vi "Apply on Cell.vi"(8 "error in":errorcluster, 10 "Cell":refnum<class "Cell.lvclass">, 11 "Cell View Alternating Back Color in":refnum<class "Cell View Alternating Back Color.lvclass">) -> (0 "error out":errorcluster, 3 "Cell View Alternating Back Color out":refnum<class "Cell View Alternating Back Color.lvclass">)   [LabVIEW 2024, in "SourceGrid.lvlib" / "Cell View Alternating Back Color.lvclass"]
uses:
  Cell View Alternating Back Color.lvclass
  Cells/Cell/Cell.lvclass
  Cell View Alternating Back Color.lvclass/Cell View Alternating Back Color.ctl
  Cells/Cell/Cell.lvclass/Cell.ctl
  Cell View/Cell View.lvclass/Cell View.ctl
  D:/git/Sourcegrid-LabVIEW/dll/SourceGrid.dll
  dll/SourceGrid.dll
  Cell View/Cell View.lvclass
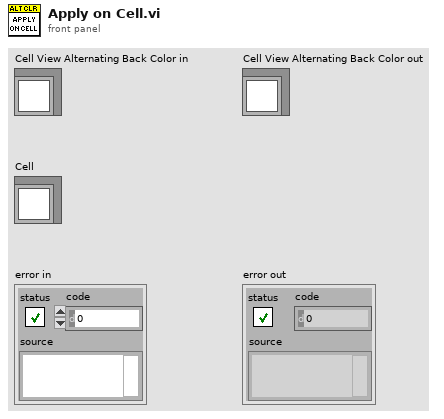
[diagram p1: front panel]
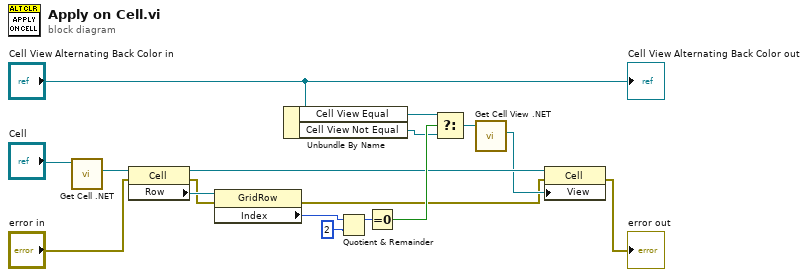
[diagram p0: block diagram]
diagram:
  n1 = call "Get Cell .NET.vi"("Cell in"="Cell") -> ("Cell .NET"=w13:refnum<k24>)  [unwired: 9 in, 1 out]
  n2 = property class="Cell"(reference=w13, error in="error in") -> (reference out=w5:refnum<k24>, error out=w11:errorcluster, "Row"=w12:refnum<k24>)
  n3 = property class="GridRow"(reference=w12, error in=w11) -> (error out=w2:errorcluster, "Index"=w9:i32)  [unwired: 1 out]
  n4 = Unbundle By Name("Cell View Alternating Back Color in") -> ("Cell View Equal"=w7:refnum<class "Cell View.lvclass">, "Cell View Not Equal"=w6:refnum<class "Cell View.lvclass">)
  n5 = Quotient & Remainder(x=w9, y=2) -> (x-y*floor(x/y)=w16:i32)  [unwired: 1 out]
  n6 = Equal To 0?(x=w16) -> (x = 0?=w15:bool)
  n7 = Select(t=w7, s=w15, f=w6) -> (s? t:f=w4:refnum<class "Cell View.lvclass">)
  n8 = call "Get Cell View .NET.vi"("Cell View in"=w4) -> ("Cell View .NET"=w3:refnum<k24>)  [unwired: 9 in, 1 out]
  n9 = property class="Cell"(reference=w5, error in=w2, "View"=w3) -> (error out=→"error out":errorcluster)  [unwired: 1 out]
  "Cell View Alternating Back Color out" <- "Cell View Alternating Back Color in"
